vi "iXonKinetic.vi"() -> ()   [LabVIEW 2009]
panel:
  in  "Shutter opens on TTL":i32(ring)=1 items=["Low", "High"]
  in  "Top":i32=128
  in  "Right":i32=128
  in  "Vertical bin":i32=1
  in  "Horizontal bin":i32=1
  in  "stop":bool
  in  "OK Button":bool
  in  "Number in series":i32=3
  in  "Scan to display":i32=1
  out "Intensity Graph":dbl[][](graph)
  out "Detector Y Pixels":i32
  in  "Time to open or\nclose shutter (ms):":i32
  out "Return from CheckTimings":u32
  out "Detector X Pixels":i32
  out "Return from GetStatus":u32
  out "Return from Start Acquisition":u32
  out "Return from GetAcquiredData":u32
  out "Calculated Exposure Value":sgl format="%.4f"
  in  "Shutter Time (secs)":sgl=0.05 format="%.4f"
  out "Return from Initialize":u32
  in  "Trigger":u32(ring) items=["Internal", "External"]
  # "Status"
  # "Acquisition Mode: Single Scan\nReadout Mode: Full Resolution Image\nOnly showing one track of data"
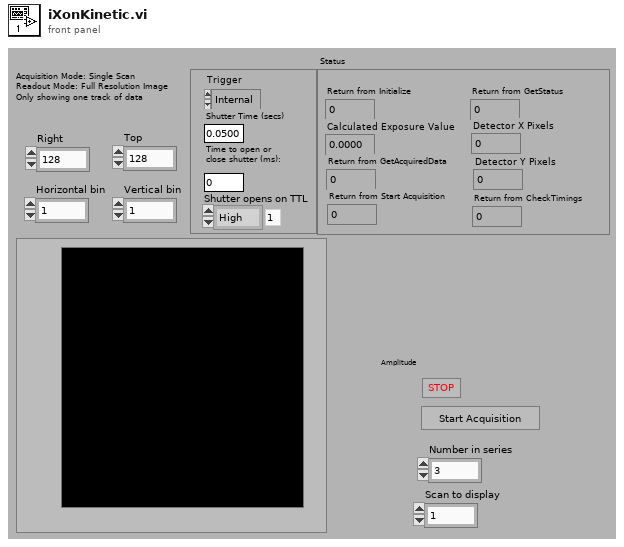
[diagram p1: front panel]
types:
  T1 = typedef "Error Code Enum typedef.ctl" = enum32{"N/A (0)", "DRV_ERROR_CODES", "DRV_SUCCESS", "DRV_VXDNOTINSTALLED", "DRV_ERROR_SCAN", "DRV_ERROR_CHECK_SUM", "DRV_ERROR_FILELOAD", "DRV_UNKNOWN_FUNC", "DRV_ERROR_VXD_INIT", "DRV_ERROR_ADDRESS", "DRV_ERROR_PAGELOCK", "DRV_ERROR_PAGEUNLOCK", "DRV_ERROR_BOARDTEST", "DRV_ERROR_ACK", "DRV_ERROR_UP_FIFO", "DRV_ERROR_PATTERN", "N/A (16)", "DRV_ACQUISITION_ERRORS", "DRV_ACQ_BUFFER", "DRV_ACQ_DOWNFIFO_FULL", "DRV_PROC_UNKONWN_INSTRUCTION", "DRV_ILLEGAL_OP_CODE", "DRV_KINETIC_TIME_NOT_MET", "DRV_ACCUM_TIME_NOT_MET", "DRV_NO_NEW_DATA", "N/A (25)", "DRV_SPOOLERROR", "N/A (27)", "N/A (28)", "N/A (29)", "N/A (30)", "N/A (31)", "N/A (32)", "DRV_TEMPERATURE_CODES", "DRV_TEMPERATURE_OFF", "DRV_TEMPERATURE_NOT_STABILIZED", "DRV_TEMPERATURE_STABILIZED", "DRV_TEMPERATURE_NOT_REACHED", "DRV_TEMPERATURE_OUT_RANGE", "DRV_TEMPERATURE_NOT_SUPPORTED", "DRV_TEMPERATURE_DRIFT", "N/A (41)", "N/A (42)", "N/A (43)", "N/A (44)", "N/A (45)", "N/A (46)", "N/A (47)", "N/A (48)", "DRV_GENERAL_ERRORS", "DRV_INVALID_AUX", "DRV_COF_NOTLOADED", "DRV_FPGAPROG", "DRV_FLEXERROR", "DRV_GPIBERROR", "N/A (55)", "N/A (56)", "N/A (57)", "N/A (58)", "N/A (59)", "N/A (60)", "N/A (61)", "N/A (62)", "N/A (63)", "DRV_DATATYPE", "DRV_DRIVER_ERRORS", "DRV_P1INVALID", "DRV_P2INVALID", "DRV_P3INVALID", "DRV_P4INVALID", "DRV_INIERROR", "DRV_COFERROR", "DRV_ACQUIRING", "DRV_IDLE", "DRV_TEMPCYCLE", "DRV_NOT_INITIALIZED", "DRV_P5INVALID", "DRV_P6INVALID", "DRV_INVALID_MODE", "DRV_INVALID_FILTER", "DRV_I2CERRORS", "DRV_I2CDEVNOTFOUND", "DRV_I2CTIMEOUT", "DRV_P7INVALID", "N/A (84)", "N/A (85)", "N/A (86)", "N/A (87)", "N/A (88)", "N/A (89)", "DRV_IOCERROR", "DRV_VRMVERSIONERROR"}
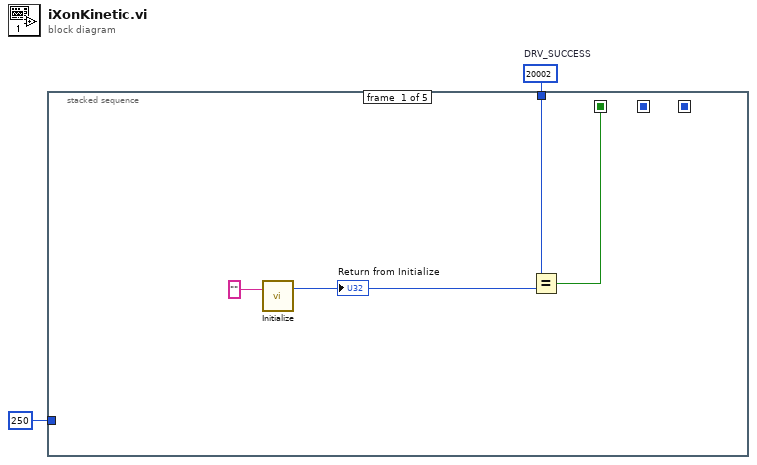
[diagram p0: block diagram]
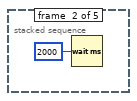
[diagram p2: hidden frame]
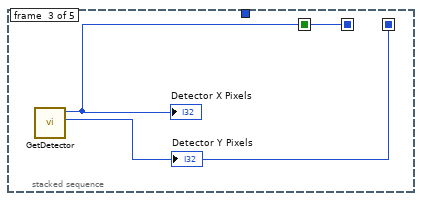
[diagram p3: hidden frame]
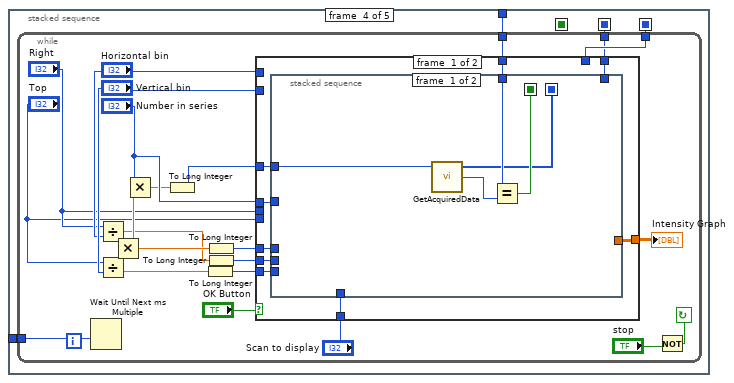
[diagram p4: hidden frame]
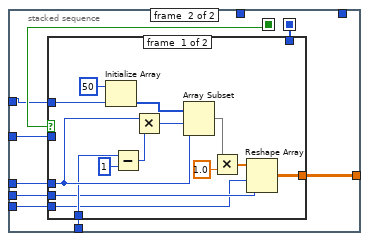
[diagram p5: hidden frame]
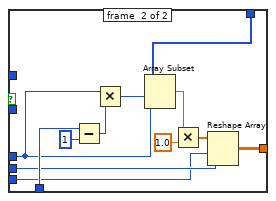
[diagram p6: hidden frame]
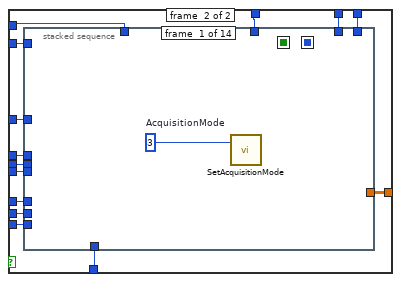
[diagram p7: hidden frame]
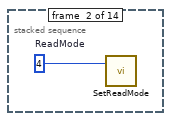
[diagram p8: hidden frame]
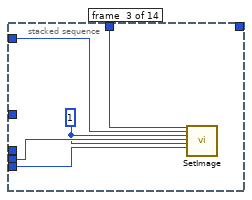
[diagram p9: hidden frame]
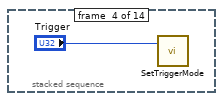
[diagram p10: hidden frame]
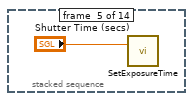
[diagram p11: hidden frame]
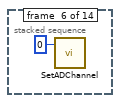
[diagram p12: hidden frame]
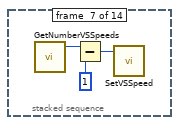
[diagram p13: hidden frame]
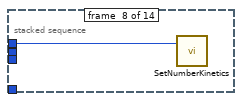
[diagram p14: hidden frame]
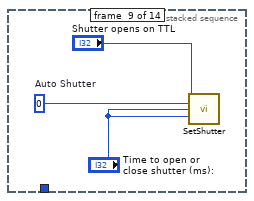
[diagram p15: hidden frame]
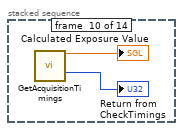
[diagram p16: hidden frame]
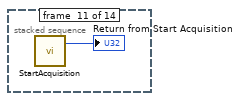
[diagram p17: hidden frame]
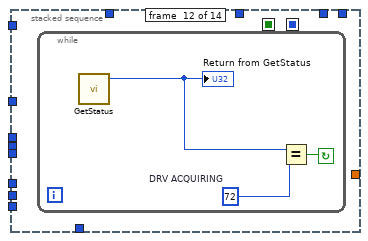
[diagram p18: hidden frame]
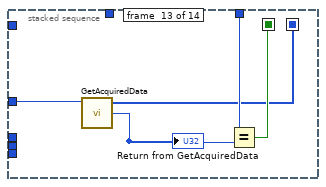
[diagram p19: hidden frame]
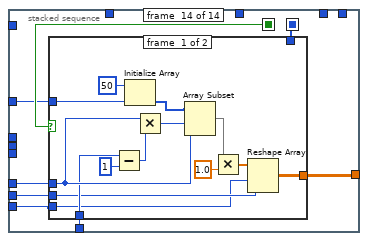
[diagram p20: hidden frame]
diagram:
  w2 = 20002  # DRV_SUCCESS
  n1 = stacked-sequence {
    seq-local: [w5 _ _ _ _] -> [_ _ _ _ w161]
    seq-local: [_ _ w9 _ _] -> [_ _ _ w13 _]
    seq-local: [_ _ w8 _ _] -> [_ _ _ w12 _]
    tunnel: w2 -> [w6 _ _ w11 _]
    tunnel: 250 -> [_ _ _ w10 _]
    frame #0 {
      n2 = call <userlib>:"Initialize.vi"("directory (\"\")"="") -> ("DLL error code"=w3:u32)  [unwired: 1 in, 1 out]
      "Return from Initialize" <- w3
      n3 = Equal?(x=w6, y=w3) -> (x = y?=w5:bool)
    }
    frame #1 {
      n4 = Wait (ms)(milliseconds to wait=u32 2000) -> ()  [unwired: 1 out]
    }
    frame #2 {
      n5 = call <userlib>:"GetDetector.vi"() -> ("ypixels"=w8:i32, "xpixels"=w9:i32)  [unwired: 4 in, 2 out]
      "Detector X Pixels" <- w9
      "Detector Y Pixels" <- w8
    }
    frame #3 {
      n6 = while {
        tunnel: w13 -> [w16]
        tunnel: w12 -> [w25]
        tunnel: w11 -> [w35]
        tunnel: w10 -> [w29]
        stop <- w32 continue-if-true
        n7 = Wait Until Next ms Multiple(millisecond multiple=w29) -> ()  [unwired: 1 out]
        n8 = Divide(x="Right", y="Horizontal bin") -> (x/y=w17:dbl)
        n9 = Divide(x="Top", y="Vertical bin") -> (x/y=w19:dbl)
        n10 = Multiply(x=w17, y=w19) -> (x*y=w20:dbl)
        n11 = Multiply(x="Number in series", y=w20) -> (x*y=w27:dbl)
        n12 = To Long Integer(number=w27) -> (32bit integer=w26:i32)
        n13 = To Long Integer(number=w19) -> (32bit integer=w21:i32)
        n14 = To Long Integer(number=w20) -> (32bit integer=w18:i32)
        n15 = To Long Integer(number=w17) -> (32bit integer=w22:i32)
        n16 = case shown="True" "OK Button" {
          tunnel: w16 -> [w44 w96]
          tunnel: [w43 w98] -> w31
          tunnel: "Scan to display" -> [w39 w97]
          tunnel: w35 -> [w42 w87]
          tunnel: "Number in series" -> [w41 w95]
          tunnel: w18 -> [w40 w94]
          tunnel: "Horizontal bin" -> [_ w92]
          tunnel: "Vertical bin" -> [_ w91]
          tunnel: w26 -> [w38 w93]
          tunnel: w21 -> [w37 w89]
          tunnel: w22 -> [w36 w88]
          tunnel: w25 -> [_ w90]
          tunnel: "Right" -> [_ w86]
          tunnel: "Top" -> [_ w85]
          frame #0 {
            n17 = stacked-sequence {
              seq-local: [w48 _] -> [_ w53]
              seq-local: [w46 _] -> [_ w55]
              tunnel: w44 -> [_ _]
              tunnel: [_ w56] -> w43
              tunnel: w42 -> [w49 _]
              tunnel: w41 -> [_ w57]
              tunnel: w40 -> [_ w54]
              tunnel: w38 -> [w47 w50]
              tunnel: w39 -> [_ w58]
              tunnel: w37 -> [_ w52]
              tunnel: w36 -> [_ w51]
              frame #0 {
                n18 = call <userlib>:"GetAcquiredData.vi"("size"=w47) -> ("DLL error code"=w45:u32, "array"=w46:i32[])  [unwired: 2 in, 1 out]
                n19 = Equal?(x=w49, y=w45) -> (x = y?=w48:bool)
              }
              frame #1 {
                n20 = case shown="False" w53 {
                  tunnel: w58 -> [w65 w78]
                  tunnel: w57 -> [_ _]
                  tunnel: [w64 w77] -> w56
                  tunnel: w55 -> [_ w76]
                  tunnel: w54 -> [w66 w75]
                  tunnel: w52 -> [w62 w73]
                  tunnel: w51 -> [w63 w74]
                  tunnel: w50 -> [w60 _]
                  frame #0 {
                    n21 = Initialize Array "Initialize Array"(50, w60) -> (w59:i32[])
                    n22 = Subtract(x=w65, y=1) -> (x-y=w69:i32)
                    n23 = Multiply(x=w66, y=w69) -> (x*y=w68:i32)
                    n24 = Array Subset(array=w59, index=w68, length=w66) -> (w67:i32[])
                    n25 = Multiply(x=w67, y=1.0) -> (x*y=w71:dbl[])
                    n26 = Reshape Array(w71, w62, w63) -> (w64:dbl[][])
                  }
                  frame #1 {
                    n27 = Subtract(x=w78, y=1) -> (x-y=w81:i32)
                    n28 = Multiply(x=w75, y=w81) -> (x*y=w80:i32)
                    n29 = Array Subset(array=w76, index=w80, length=w75) -> (w79:i32[])
                    n30 = Multiply(x=w79, y=1.0) -> (x*y=w83:dbl[])
                    n31 = Reshape Array(w83, w73, w74) -> (w77:dbl[][])
                  }
                }
              }
            }
          }
          frame #1 {
            n32 = stacked-sequence {
              seq-local: [_ _ _ _ _ _ _ _ _ _ _ _ w125 _] -> [_ _ _ _ _ _ _ _ _ _ _ _ _ w134]
              seq-local: [_ _ _ _ _ _ _ _ _ _ _ _ w123 _] -> [_ _ _ _ _ _ _ _ _ _ _ _ _ w129]
              tunnel: w96 -> [_ _ _ _ _ _ _ _ _ _ _ _ _ _]
              tunnel: [_ _ _ _ _ _ _ _ _ _ _ _ _ w128] -> w98
              tunnel: w97 -> [_ _ _ _ _ _ _ _ _ _ _ _ _ w130]
              tunnel: w95 -> [_ _ _ _ _ _ _ w112 _ _ _ _ _ _]
              tunnel: w94 -> [_ _ _ _ _ _ _ _ _ _ _ _ _ w133]
              tunnel: w93 -> [_ _ _ _ _ _ _ _ _ _ _ _ w124 w127]
              tunnel: w92 -> [_ _ w105 _ _ _ _ _ _ _ _ _ _ _]
              tunnel: w91 -> [_ _ w104 _ _ _ _ _ _ _ _ _ _ _]
              tunnel: w90 -> [_ _ _ _ _ _ _ _ _ _ _ _ _ _]
              tunnel: w89 -> [_ _ _ _ _ _ _ _ _ _ _ _ _ w131]
              tunnel: w88 -> [_ _ _ _ _ _ _ _ _ _ _ _ _ w132]
              tunnel: w87 -> [_ _ _ _ _ _ _ _ _ _ _ _ w126 _]
              tunnel: w86 -> [_ _ w103 _ _ _ _ _ _ _ _ _ _ _]
              tunnel: w85 -> [_ _ w101 _ _ _ _ _ _ _ _ _ _ _]
              frame #0 {
                w99 = u16 3  # AcquisitionMode
                n33 = call <userlib>:"SetAcquisitionMode.vi"("mode"=w99) -> ()  [unwired: 1 in, 2 out]
              }
              frame #1 {
                w100 = u16 4  # ReadMode
                n34 = call <userlib>:"SetReadMode.vi"("mode"=w100) -> ()  [unwired: 1 in, 2 out]
              }
              frame #2 {
                w102 = 1
                n35 = call <userlib>:"SetImage.vi"("hbin"=w105, "vbin"=w104, "hstart"=w102, "hend"=w103, "vstart"=w102, "vend"=w101) -> ()  [unwired: 20 in, 2 out]
              }
              frame #3 {
                n36 = call <userlib>:"SetTriggerMode.vi"("mode"="Trigger") -> ()  [unwired: 1 in, 2 out]
              }
              frame #4 {
                n37 = call <userlib>:"SetExposureTime.vi"("time"="Shutter Time (secs)") -> ()  [unwired: 1 in, 2 out]
              }
              frame #5 {
                n38 = call <userlib>:"SetADChannel.vi"("channel"=0) -> ()  [unwired: 1 in, 2 out]
              }
              frame #6 {
                n39 = call <userlib>:"GetNumberVSSpeeds.vi"() -> ("number"=w111:i32)  [unwired: 3 in, 2 out]
                n40 = Subtract(x=w111, y=1) -> (x-y=w109:i32)
                n41 = call <userlib>:"SetVSSpeed.vi"("index"=w109) -> ()  [unwired: 1 in, 2 out]
              }
              frame #7 {
                n42 = call <userlib>:"SetNumberKinetics.vi"("number"=w112) -> ()  [unwired: 1 in, 2 out]
              }
              frame #8 {
                w114 = 0  # Auto Shutter
                n43 = call <userlib>:"SetShutter.vi"("type"="Shutter opens on TTL", "mode"=w114, "closingtime"="Time to open or\nclose shutter (ms):", "openingtime"="Time to open or\nclose shutter (ms):") -> ()  [unwired: 10 in, 2 out]
              }
              frame #9 {
                n44 = call <userlib>:"GetAcquisitionTimings.vi"() -> ("exposure"=→"Calculated Exposure Value":sgl, "DLL error code"=→"Return from CheckTimings":u32)  [unwired: 11 in, 3 out]
              }
              frame #10 {
                n45 = call <userlib>:"StartAcquisition.vi"() -> ("DLL error code"=→"Return from Start Acquisition":u32)  [unwired: 2 in, 1 out]
              }
              frame #11 {
                n46 = while {
                  stop <- w120 continue-if-true
                  w121 = u16 72  # DRV ACQUIRING
                  n47 = call <userlib>:"GetStatus.vi"() -> ("status"=w119:T1)  [unwired: 3 in, 2 out]
                  "Return from GetStatus" <- w119
                  n48 = Equal?(x=w119, y=w121) -> (x = y?=w120:bool)
                }
              }
              frame #12 {
                n49 = call <userlib>:"GetAcquiredData.vi"("size"=w124) -> ("DLL error code"=w122:u32, "array"=w123:i32[])  [unwired: 2 in, 1 out]
                "Return from GetAcquiredData" <- w122
                n50 = Equal?(x=w126, y=w122) -> (x = y?=w125:bool)
              }
              frame #13 {
                n51 = case shown="False" w134 {
                  tunnel: w130 -> [w141 w155]
                  tunnel: [w140 w154] -> w128
                  tunnel: w129 -> [_ w153]
                  tunnel: w133 -> [w142 w152]
                  tunnel: w131 -> [w138 w150]
                  tunnel: w132 -> [w139 w151]
                  tunnel: w127 -> [w136 _]
                  frame #0 {
                    n52 = Subtract(x=w141, y=1) -> (x-y=w145:i32)
                    n53 = Initialize Array "Initialize Array"(50, w136) -> (w135:i32[])
                    n54 = Multiply(x=w142, y=w145) -> (x*y=w144:i32)
                    n55 = Array Subset(array=w135, index=w144, length=w142) -> (w143:i32[])
                    n56 = Multiply(x=w143, y=1.0) -> (x*y=w147:dbl[])
                    n57 = Reshape Array(w147, w138, w139) -> (w140:dbl[][])
                  }
                  frame #1 {
                    n58 = Subtract(x=w155, y=1) -> (x-y=w157:i32)
                    n59 = Multiply(x=w152, y=w157) -> (x*y=w156:i32)
                    n60 = Array Subset(array=w153, index=w156, length=w152) -> (w149:i32[])
                    n61 = Multiply(x=w149, y=1.0) -> (x*y=w159:dbl[])
                    n62 = Reshape Array(w159, w150, w151) -> (w154:dbl[][])
                  }
                }
              }
            }
          }
        }
        "Intensity Graph" <- w31
        n63 = Not(x="stop") -> (.not. x?=w32:bool)
      }
    }
    frame #4 {
      n64 = case shown="True" w161 {
        frame #0 {
        }
        frame #1 {
          n65 = call <userlib>:"ShutDown.vi"() -> ()  [unwired: 2 in, 2 out]
        }
      }
    }
  }
